vi "testing_SPI.vi"() -> ()   [LabVIEW 2009]
panel:
  out "total cycles":i32
  out "bucle":i32
  out "error quantity":i32
  out "data read value":u32
  out "error out 2":errorcluster
  in  "error in (no error)":errorcluster
  out "data":u32
  out "hex integer string":string
  out "Id in":i32=72
  in  "Read physical":bool
  out "Data to send hex":string
  in  "Device":u16(ring) items=["Attenuation", "Clipping", "Enable channel", "Delay line", "ASIC"]
  in  "Read/#write":bool
  out "data out serial":string
  in  "stop":bool
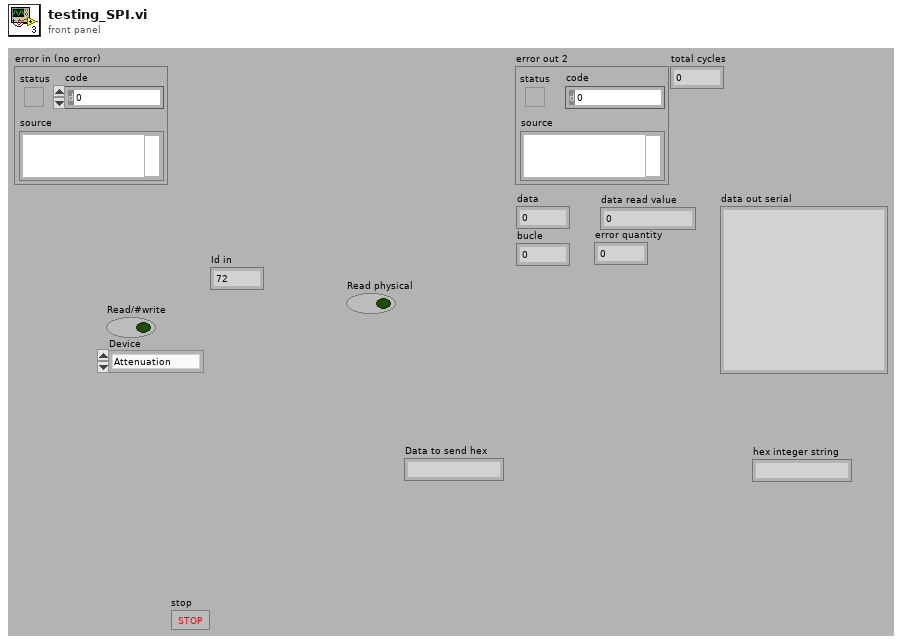
[diagram p1: front panel]
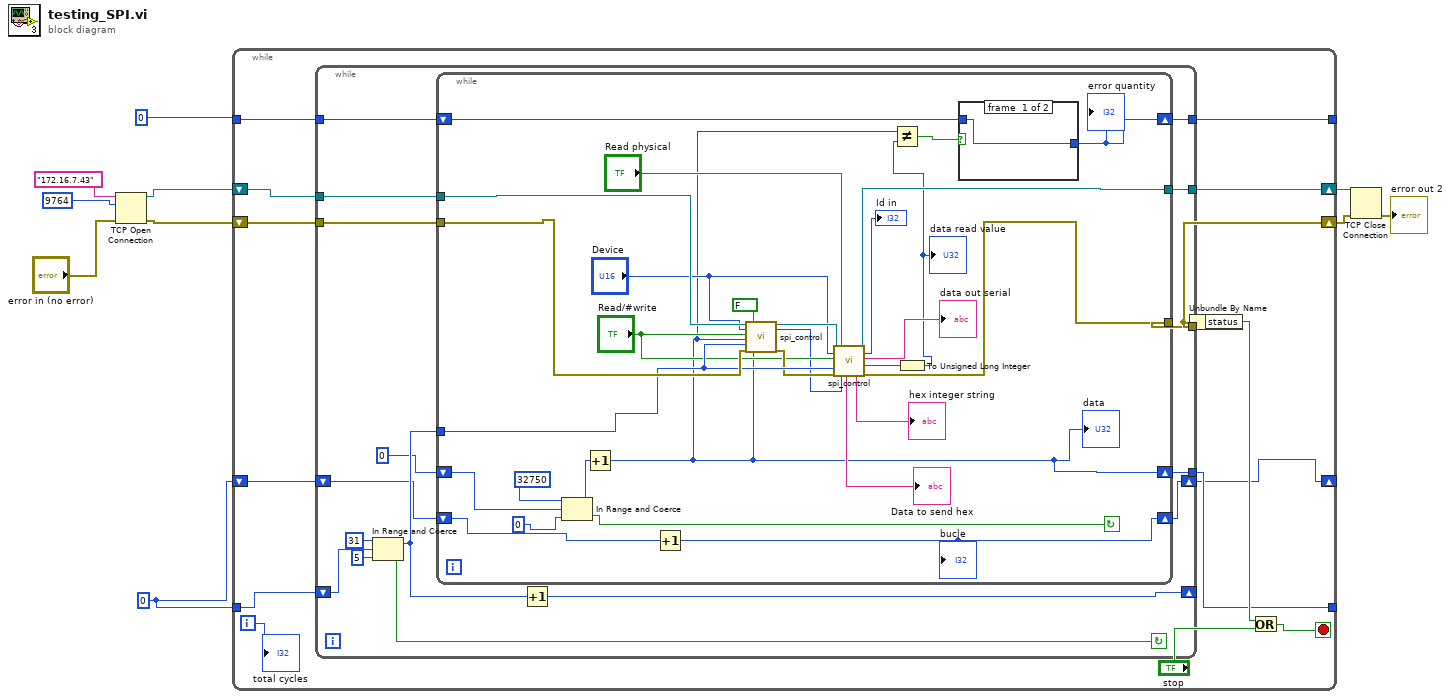
[diagram p0: block diagram]
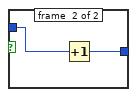
[diagram p2: hidden frame]
diagram:
  w1 = 0 ("lower limit")
  n1 = TCP Open Connection(address="172.16.7.43", remote port or service name=u16 9764, error in (no error)="error in (no error)") -> (connection ID=w6:refnum<k5>, error out=w5:errorcluster)  [unwired: 2 in]
  n2 = while {
    shift-right: [w24] -> w8
    shift-left: w5 -> [w19]
    shift-right: [w17] -> w7
    shift-left: w6 -> [w20]
    tunnel: 0 ("lower limit") -> [w15]
    tunnel: [w14] -> _
    tunnel: w1 -> [w16]
    tunnel: [w18] -> _
    shift-right: [w12] -> _
    shift-left: w1 -> [w13]
    i -> [w11]
    stop <- w23 stop-if-true
    n3 = while {
      tunnel: [w40] -> w24
      tunnel: w20 -> [w39]
      tunnel: w19 -> [w38]
      tunnel: [w37] -> w18
      tunnel: [w36] -> w17
      shift-right: [w31] -> _
      shift-left: w16 -> [w33]
      tunnel: w15 -> [w28]
      tunnel: [w27] -> w14
      shift-right: [w25] -> w12
      shift-left: w13 -> [w26]
      stop <- w30 continue-if-true
      n4 = In Range and Coerce(upper limit=31, x=w33, lower limit=5) -> (coerced(x)=w32:i32, In Range?=w30:bool)
      n5 = while {
        tunnel: [w69] -> w40
        tunnel: w39 -> [w68]
        tunnel: w38 -> [w67]
        tunnel: [w66] -> w36
        shift-right: [w45] -> w37
        shift-left: u32 0 -> [w64]
        tunnel: w32 -> [w60]
        shift-right: [w47] -> w27
        shift-left: w28 -> [w48]
        shift-right: [w43] -> w25
        shift-left: w26 -> [w44]
        stop <- w61 continue-if-true
        n6 = In Range and Coerce(upper limit=u32 32750, x=w64, lower limit=u32 0) -> (coerced(x)=w65:u32, In Range?=w61:bool)
        n7 = Increment(x=w65) -> (x+1=w45:u32)
        "data" <- w45
        n8 = Increment(x=w44) -> (x+1=w43:i32)
        "bucle" <- w43
        n9 = call "spi_control.vi"("connection ID"=w68, "Device"="Device", "Read/#write"="Read/#write", "Data"=w45, "Register or channel"=w60, "error out 3"=w67, "Read physical"=FALSE, "Id in"=w45) -> ("connection ID out"=w51:refnum<k5>, "Id out"=w49:i32, "error out 2"=w54:errorcluster)  [unwired: 4 in, 5 out]
        n10 = call "spi_control.vi"("connection ID"=w51, "Device"="Device", "Read/#write"="Read/#write", "Register or channel"=w60, "error out 3"=w54, "Read physical"="Read physical", "Id in"=w49) -> ("Data to send hex"=→"Data to send hex":string, "hex integer string"=→"hex integer string":string, "connection ID out"=w66:refnum<k5>, "Id out"=→"Id in":i32, "data out serial"=→"data out serial":string, "data read value"=w41:u32, "error out 2"=w69:errorcluster)  [unwired: 5 in, 1 out]
        n11 = To Unsigned Long Integer(number=w41) -> (unsigned 32bit integer=w42:u32)
        "data read value" <- w42
        n12 = Not Equal?(x=w45, y=w42) -> (x != y?=w46:bool)
        n13 = case shown="True" w46 {
          tunnel: w48 -> [w70 w72]
          tunnel: [w70 w71] -> w47
          frame #0 {
          }
          frame #1 {
            n14 = Increment(x=w72) -> (x+1=w71:i32)
          }
        }
        "error quantity" <- w47
      }
      n15 = Increment(x=w32) -> (x+1=w31:i32)
    }
    n16 = Unbundle By Name(w24) -> ("status"=w22:bool)
    n17 = Or(x=w22, y="stop") -> (x .or. y?=w23:bool)
    "total cycles" <- w11
  }
  n18 = TCP Close Connection(connection ID=w7, error in (no error)=w8) -> (error out=→"error out 2":errorcluster)  [unwired: 1 in, 1 out]
